vi "Master Setup Prompt.vi"(7 "Master Setup File (in)":path) -> (2 "Current File Paths":path[](array[path]), 3 "Master Setup File (out)":path)   [LabVIEW 2017]
panel:
  in  "Auto Correct":bool
  in  "Continue":bool
  in  "Clear Files":bool
  in  "Clear":bool[](array[boolean])
  out "Setup Description":string[](array[string])
  in  "Browse":bool[](array[boolean])
  in  "Select Directory":bool
  in  "Cancel":bool
  in  "OK":bool
  out "Status":u16[](array[ring])
  out "Old File Paths":path[](array[path])
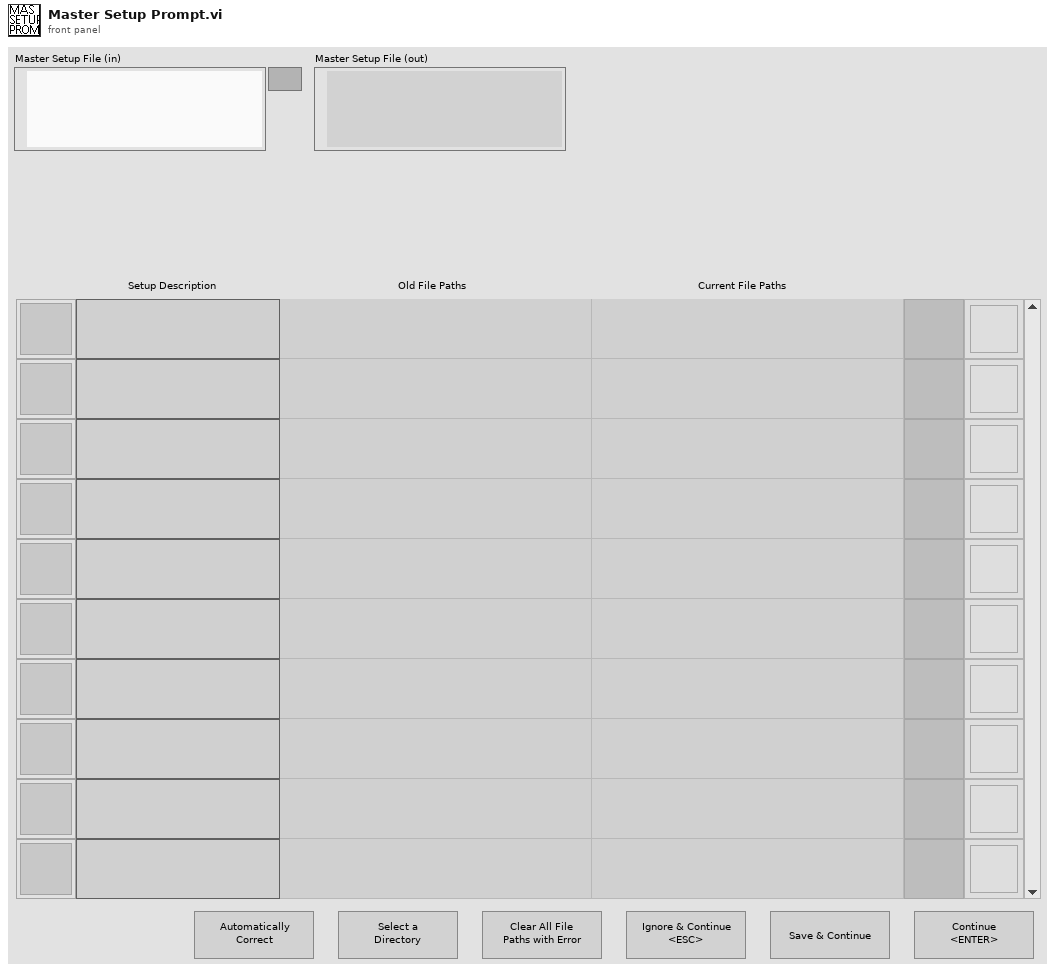
[diagram p1: front panel]
types:
  T1 = enum16{"Initialize", "Load Master Setup", "Check if Files Exist", "Idle", "Automatically Correct", "Browse for Directory", "Clear Files with Error", "Browse for File", "Clear Selected File", "Save Changes"}
  T2 = enum16{"open", "replace", "create", "open or create", "replace or create", "replace or create with confirmation"}
  T3 = enum16{"Initialize", "Load Master Setup", "Check if Files Exist", "Idle", "Automatically Correct", "Browse for Directory", "Clear Files with Error", "Browse for File", "Clear Selected File", "Save Changes"}[]
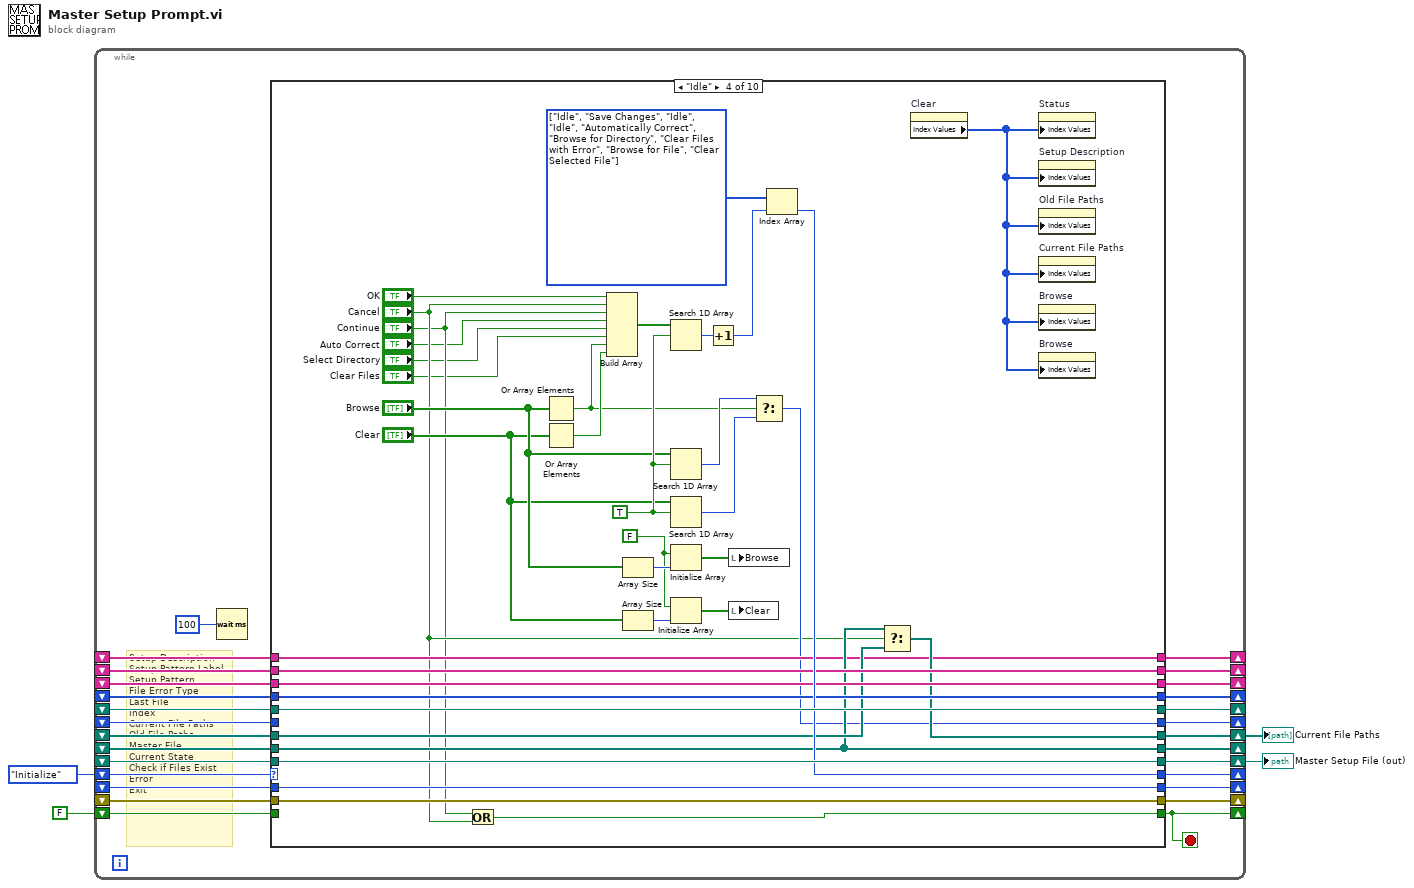
[diagram p0: block diagram]
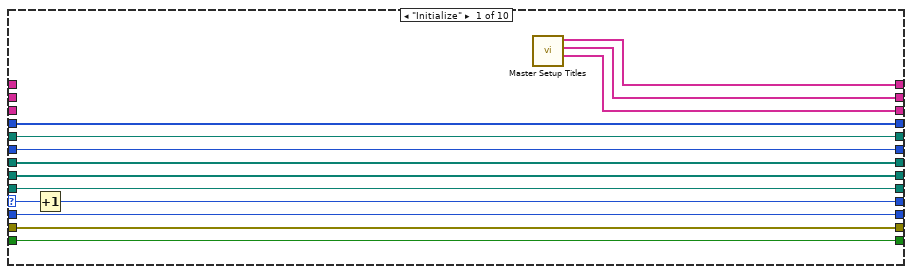
[diagram p2: hidden frame]
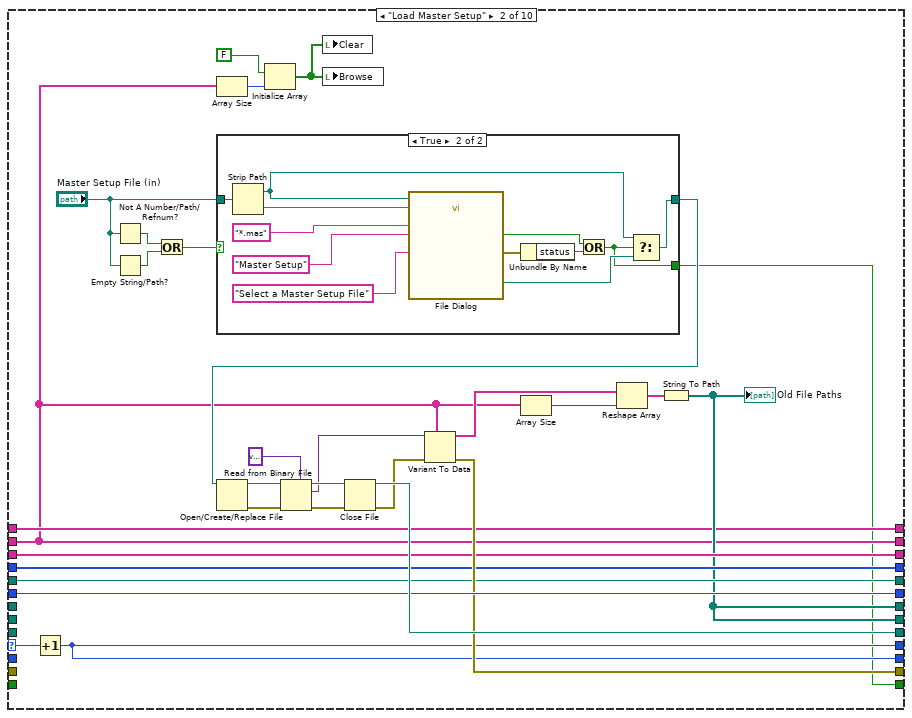
[diagram p3: hidden frame]
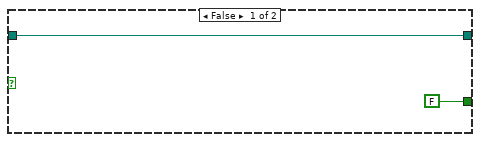
[diagram p4: hidden frame]
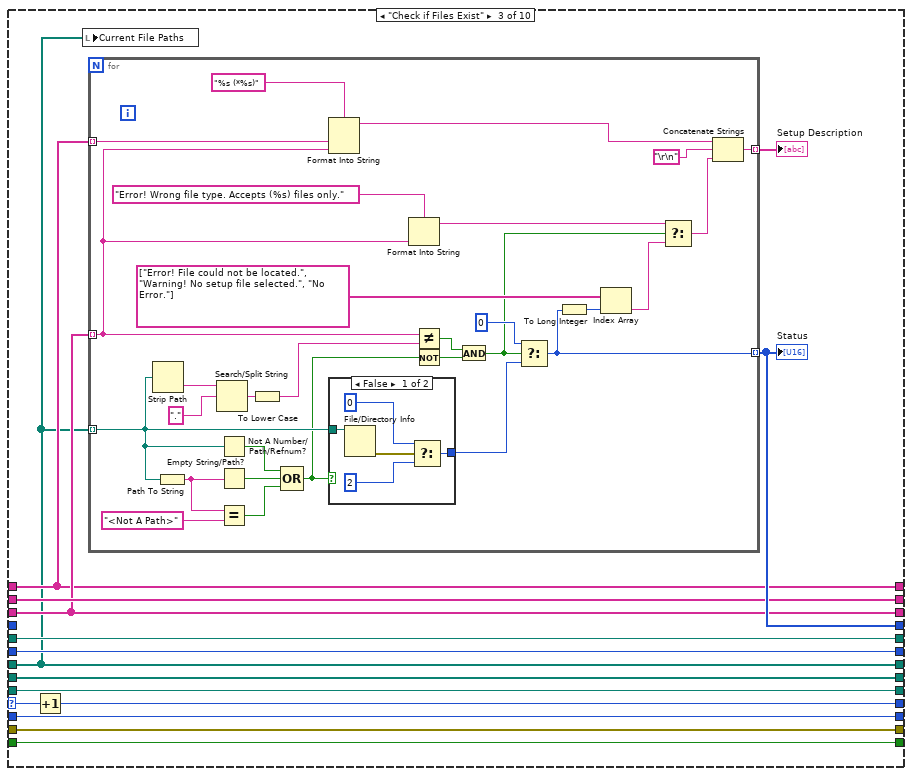
[diagram p5: hidden frame]
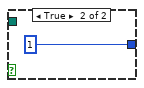
[diagram p6: hidden frame]
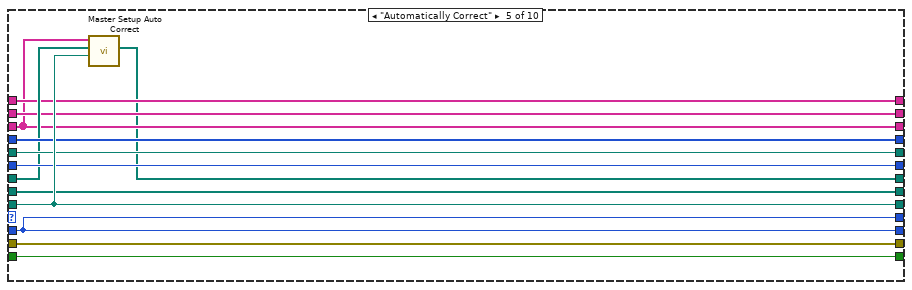
[diagram p7: hidden frame]
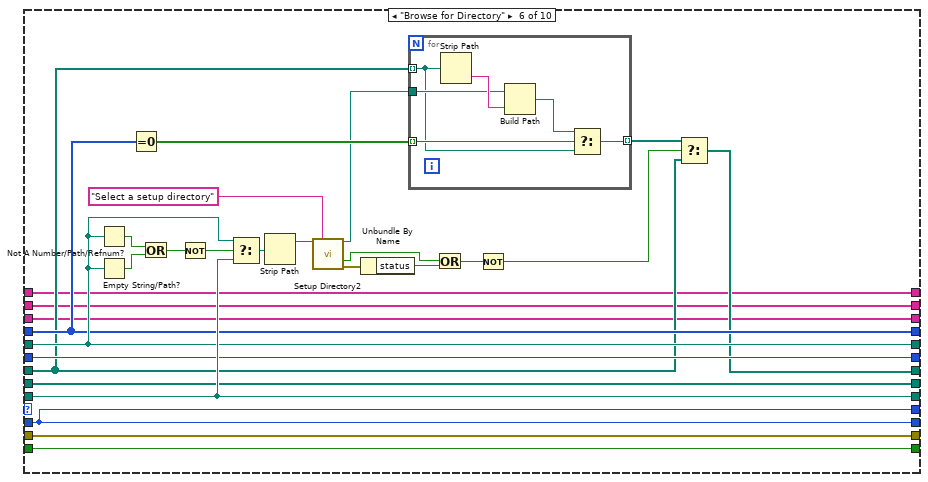
[diagram p8: hidden frame]
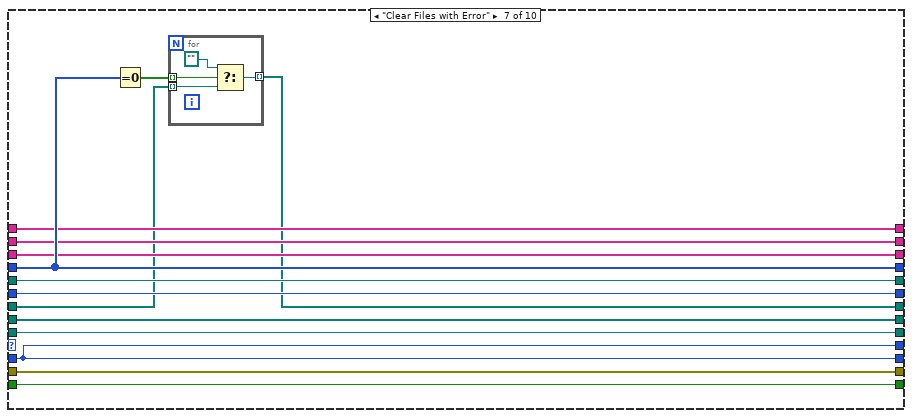
[diagram p9: hidden frame]
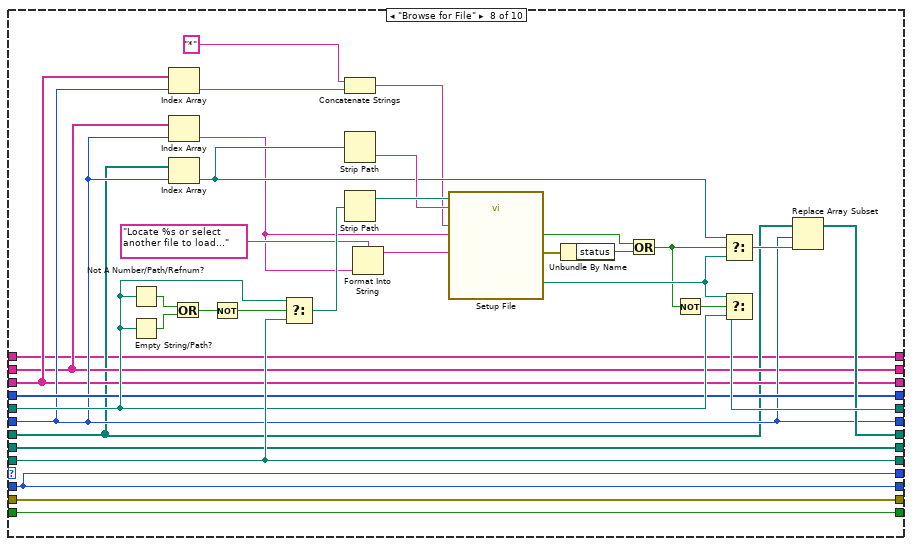
[diagram p10: hidden frame]
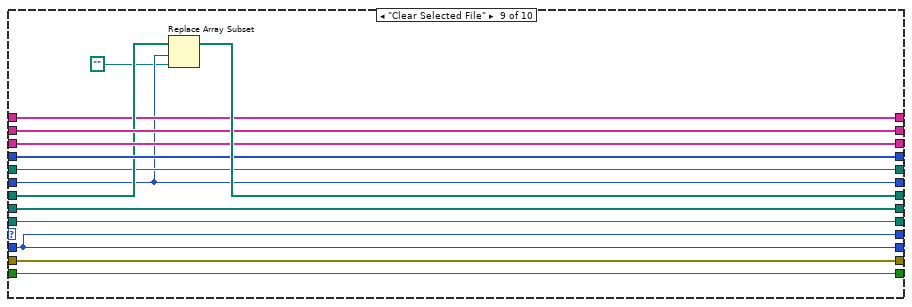
[diagram p11: hidden frame]
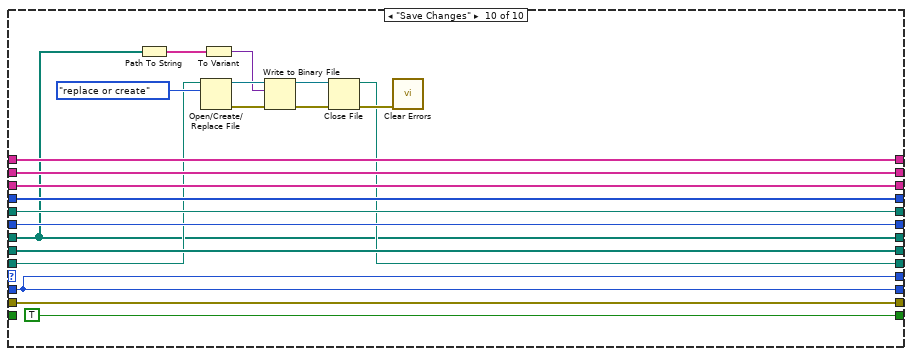
[diagram p12: hidden frame]
diagram:
  n1 = while {
    shift-right: [w21] -> _
    shift-left: FALSE -> [w25]
    shift-right: [w30] -> w3
    shift-left: _ -> [w31]
    shift-right: [w28] -> _
    shift-left: _ -> [w29]
    shift-right: [w26] -> w2
    shift-left: _ -> [w27]
    shift-right: [w18] -> _
    shift-left: T1."Initialize" -> [w24]
    shift-right: [w22] -> _
    shift-left: _ -> [w23]
    shift-right: [w19] -> _
    shift-left: _ -> [w20]
    shift-right: [w16] -> _
    shift-left: _ -> [w17]
    shift-right: [w13] -> _
    shift-left: _ -> [w14]
    shift-right: [w9] -> _
    shift-left: _ -> [w12]
    shift-right: [w10] -> _
    shift-left: _ -> [w11]
    shift-right: [w7] -> _
    shift-left: _ -> [w8]
    shift-right: [w5] -> _
    shift-left: _ -> [w6]
    stop <- w21 stop-if-true
    # "Setup Description\nSetup Pattern Label\nSetup Pattern\nFile Error Type\nLast File\nIndex\nCurrent File Paths\nOld File Paths\nMaster File\nCurrent State\nCheck if Files Exist\nError\nExit"
    n2 = Wait (ms)(milliseconds to wait=u32 100) -> ()  [unwired: 1 out]
    n3 = case shown="\"Idle\"" w24 {
      selector: w24 -> [w42 w64 w101 _ _ _ _ _ _ _]
      tunnel: w25 -> [w45 _ w100 _ w187 w206 w235 w257 w288 _]
      tunnel: w31 -> [w41 _ w103 w175 w188 w208 w236 w266 w289 w294]
      tunnel: [w45 w47 w100 w145 w187 w206 w235 w257 w288 TRUE] -> w21
      tunnel: [w41 w71 w103 w175 w188 w208 w236 w266 w289 w293] -> w30
      tunnel: w29 -> [w44 _ w104 w176 w189 w217 w237 w276 w290 w311]
      tunnel: [w44 w66 w104 w176 w189 w217 w237 w276 w290 w311] -> w28
      tunnel: w27 -> [w40 _ w90 w163 w182 w195 w225 w246 w282 w292]
      tunnel: [w40 w58 w90 w161 w177 w194 w224 w254 w286 w292] -> w26
      tunnel: w23 -> [w39 w67 w99 _ w185 w204 w233 w251 w278 w310]
      tunnel: [w36 w63 w98 w169 w186 w205 w234 w256 w287 w309] -> w18
      tunnel: [w39 w67 w99 w156 w185 w204 w233 w251 w278 w310] -> w22
      tunnel: w20 -> [w38 w65 w102 w174 w184 w202 w232 w262 w279 w308]
      tunnel: [w38 w65 w102 w174 w184 w202 w232 w255 w279 w308] -> w19
      tunnel: w17 -> [w43 _ w97 w168 w186 w205 w234 w256 w287 w309]
      tunnel: [w43 w63 w97 w168 w186 w205 w234 w256 w287 w309] -> w16
      tunnel: w14 -> [w37 w60 _ w166 w183 w201 w231 w252 w285 w306]
      tunnel: [w37 w60 w96 w166 w183 w201 w231 w252 w285 w306] -> w13
      tunnel: w12 -> [_ w59 w93 w165 w178 w192 w228 w248 w284 w305]
      tunnel: w11 -> [_ w49 w95 w164 w181 w193 w229 w247 w283 w304]
      tunnel: [w33 w49 w95 w164 w181 w193 w229 w247 w283 w304] -> w10
      tunnel: [w32 w59 w93 w165 w178 w192 w228 w248 w284 w305] -> w9
      tunnel: w8 -> [w35 _ w94 w162 w180 w191 w227 w245 w281 w303]
      tunnel: [w35 w58 w94 w162 w180 w191 w227 w245 w281 w303] -> w7
      tunnel: w6 -> [_ w52 w92 w160 w179 w190 w226 w244 w280 w302]
      tunnel: [w34 w52 w92 w160 w179 w190 w226 w244 w280 w302] -> w5
      frame "Initialize" {
        n4 = Increment(x=w42) -> (x+1=w36:T1)
        n5 = call "Master Setup Titles.vi"() -> ("Setup Patterns"=w32:string[], "Setup Description"=w33:string[], "Setup Description w/Numbers"=w34:string[])  [unwired: 6 in, 3 out]
      }
      frame "Load Master Setup" {
        n6 = Increment(x=w64) -> (x+1=w63:T1)
        n7 = Not A Number/Path/Refnum?(number/path/refnum="Master Setup File (in)") -> (NaN/Path/Refnum?=w57:bool)
        n8 = Empty String/Path?(string/path="Master Setup File (in)") -> (empty?=w56:bool)
        n9 = Or(x=w57, y=w56) -> (x .or. y?=w55:bool)
        n10 = Array Size(array=w49) -> (size(s)=w62:i32)
        n11 = case shown="True" w55 {
          tunnel: "Master Setup File (in)" -> [w77 w89]
          tunnel: [w77 w80] -> w53
          tunnel: [FALSE w79] -> w47
          frame False {
          }
          frame True {
            n12 = Strip Path(path=w89) -> (stripped path=w78:path, name=w88:string)
            n13 = call "File Dialog"("start path"=w78, "prompt"="Select a Master Setup File", "default name"=w88, "pattern (all files)"="*.mas", "pattern label"="Master Setup") -> ("selected path"=w81:path, "cancelled"=w82:bool, "error out"=w84:errorcluster)  [unwired: 7 in, 1 out]
            n14 = Unbundle By Name(w84) -> ("status"=w83:bool)
            n15 = Or(x=w82, y=w83) -> (x .or. y?=w79:bool)
            n16 = Select(t=w78, s=w79, f=w81) -> (s? t:f=w80:path)
          }
        }
        n17 = Open/Create/Replace File(file path (use dialog)=w53) -> (refnum out=w73:refnum<file>, error out=w75:errorcluster)  [unwired: 5 in, 1 out]
        n18 = Initialize Array(FALSE, w62) -> (w46:bool[])
        n19 = Read from Binary File(5:variant ("Data (in)"), 8:w75, 11:w73) -> (0:w74:errorcluster, 2:w69:variant, 3:w72:refnum<file>)  [unwired: 3 in, 1 out]
        n20 = local write "Clear"(w46) -> ()
        n21 = local write "Browse"(w46) -> ()
        n22 = Close File(refnum=w72, error in=w74) -> (path=w71:path, error out=w68:errorcluster)
        n23 = Variant To Data(error in=w68, type=w49, Variant=w69) -> (data=w51:string[], error out=w66:errorcluster)
        n24 = Array Size(array=w49) -> (size(s)=w50:i32)
        n25 = Reshape Array(w51, w50) -> (w48:string[])
        n26 = String To Path(string=w48) -> (path=w58:path[])
        "Old File Paths" <- w58
      }
      frame "Check if Files Exist" {
        n27 = Increment(x=w101) -> (x+1=w98:T1)
        n28 = local write "Current File Paths"(w90) -> ()
        n29 = for {
          tunnel: w90 -> [w128] mode=indexing
          tunnel: [w122] -> w96 mode=indexing
          tunnel: w93 -> [w106] mode=indexing
          tunnel: w92 -> [w108] mode=indexing
          tunnel: [w116] -> w91 mode=indexing
          n30 = Strip Path(path=w128) -> (name=w127:string)  [unwired: 1 out]
          n31 = Path To String(path=w128) -> (string=w131:string)
          n32 = Search/Split String(string=w127, search string/char (-)=".") -> (match + rest of string=w117:string)  [unwired: 1 in, 2 out]
          n33 = Not A Number/Path/Refnum?(number/path/refnum=w128) -> (NaN/Path/Refnum?=w132:bool)
          n34 = Empty String/Path?(string/path=w131) -> (empty?=w133:bool)
          n35 = Equal?(x=w131, y="<Not A Path>") -> (x = y?=w129:bool)
          n36 = To Lower Case(string=w117) -> (all lower case string=w109:string)
          n37 = Compound Arithmetic op=OR(w132, w133, w129) -> (w111:bool)
          n38 = Format Into String(format string="%s (*%s)" ("search string/char (-)"), w108, w106) -> (resulting string=w107:string)  [unwired: 2 in, 1 out]
          n39 = case shown="False" w111 {
            tunnel: w128 -> [w138 _]
            tunnel: [w134 u16 1] -> w125
            frame False {
              n40 = File/Directory Info(path=w138) -> (error out=w137:errorcluster)  [unwired: 1 in, 6 out]
              n41 = Select(t=u16 0, s=w137, f=u16 2) -> (s? t:f=w134:u16)
            }
            frame True {
            }
          }
          n42 = Format Into String(format string="Error! Wrong file type. Accepts (%s) files only.", w106) -> (resulting string=w119:string)  [unwired: 2 in, 1 out]
          n43 = Not Equal?(x=w106, y=w109) -> (x != y?=w112:bool)
          n44 = Not(x=w111) -> (.not. x?=w110:bool)
          n45 = And(x=w112, y=w110) -> (x .and. y?=w113:bool)
          n46 = Select(t=u16 0, s=w113, f=w125) -> (s? t:f=w122:u16)
          n47 = To Long Integer(number=w122) -> (32bit integer=w121:i32)
          n48 = Index Array(array=string[] ["Error! File could not be located.", "Warning! No setup file selected.", "No Error."], index=w121) -> (element=w120:string)
          n49 = Select(t=w119, s=w113, f=w120) -> (s? t:f=w115:string)
          n50 = Concatenate Strings(w107, "\r\n", w115) -> (w116:string)
        }
        "Status" <- w96
        "Setup Description" <- w91
      }
      frame "Idle" {
        w147 = T3 [enum."Idle", enum."Save Changes", enum."Idle", enum."Idle", enum."Automatically Correct", enum."Browse for Directory", enum."Clear Files with Error", enum."Browse for File", enum."Clear Selected File"] items=["Initialize", "Load Master Setup", "Check if Files Exist", "Idle", "Automatically Correct", "Browse for Directory", "Clear Files with Error", "Browse for File", "Clear Selected File", "Save Changes"]
        w152 = FALSE
        w159 = TRUE ("element")
        n51 = Or(x="Continue", y="Cancel") -> (x .or. y?=w145:bool)
        n52 = Or Array Elements(Boolean array="Browse") -> (logical OR=w148:bool)
        n53 = Or Array Elements(Boolean array="Clear") -> (logical OR=w149:bool)
        n54 = Build Array("OK", "Cancel", "Continue", "Auto Correct", "Select Directory", "Clear Files", w148, w149) -> (w172:bool[])
        n55 = Array Size(array="Browse") -> (size(s)=w154:i32)
        n56 = Array Size(array="Clear") -> (size(s)=w153:i32)
        n57 = Search 1D Array(1D array=w172, element=w159) -> (index of element=w171:i32)  [unwired: 1 in]
        n58 = Search 1D Array(1D array="Browse", element=w159) -> (index of element=w158:i32)  [unwired: 1 in]
        n59 = Search 1D Array(1D array="Clear", element=w159) -> (index of element=w157:i32)  [unwired: 1 in]
        n60 = Initialize Array(w152, w154) -> (w167:bool[])
        n61 = Initialize Array(w152, w153) -> (w150:bool[])
        n62 = Increment(x=w171) -> (x+1=w170:i32)
        n63 = local write "Browse"(w167) -> ()
        n64 = local write "Clear"(w150) -> ()
        n65 = Select(t=w158, s=w148, f=w157) -> (s? t:f=w156:i32)
        n66 = Index Array(array=w147, index=w170) -> (element=w169:T1)
        n67 = Select(t=w162, s="Cancel", f=w163) -> (s? t:f=w161:path[])
        n68 = property on="Clear" class="Arr"() -> ("Index Values"=w146:u32[])  [unwired: 2 in, 2 out]
        n69 = property on="Status" class="Arr (strict)"("Index Values"=w146) -> ()  [unwired: 2 in, 2 out]
        n70 = property on="Setup Description" class="Arr (strict)"("Index Values"=w146) -> ()  [unwired: 2 in, 2 out]
        n71 = property on="Old File Paths" class="Arr (strict)"("Index Values"=w146) -> ()  [unwired: 2 in, 2 out]
        n72 = property on="Current File Paths" class="Arr (strict)"("Index Values"=w146) -> ()  [unwired: 2 in, 2 out]
        n73 = property on="Browse" class="Arr"("Index Values"=w146) -> ()  [unwired: 2 in, 2 out]
        n74 = property on="Browse" class="Arr"("Index Values"=w146) -> ()  [unwired: 2 in, 2 out]
      }
      frame "Automatically Correct" {
        n75 = call "Master Setup Auto Correct.vi"("Master File Path"=w188, "Current File Paths (in)"=w182, "Setup Patterns"=w178) -> ("Current File Paths (out)"=w177:path[])  [unwired: 8 in]
      }
      frame "Browse for Directory" {
        n76 = Not A Number/Path/Refnum?(number/path/refnum=w202) -> (NaN/Path/Refnum?=w212:bool)
        n77 = Empty String/Path?(string/path=w202) -> (empty?=w211:bool)
        n78 = Equal To 0?(x=w201) -> (x = 0?=w200:bool[])
        n79 = Or(x=w212, y=w211) -> (x .or. y?=w210:bool)
        n80 = Not(x=w210) -> (.not. x?=w209:bool)
        n81 = Select(t=w202, s=w209, f=w208) -> (s? t:f=w207:path)
        n82 = Strip Path(path=w207) -> (stripped path=w216:path)  [unwired: 1 out]
        n83 = call "Setup Directory2"("start path"=w216, "prompt"="Select a setup directory") -> ("selected path"=w199:path, "cancelled"=w213:bool, "error out"=w215:errorcluster)  [unwired: 10 in, 1 out]
        n84 = Unbundle By Name(w215) -> ("status"=w214:bool)
        n85 = for {
          tunnel: w200 -> [w223] mode=indexing
          tunnel: w195 -> [w219] mode=indexing
          tunnel: w199 -> [w221]
          tunnel: [w218] -> w196 mode=indexing
          n86 = Strip Path(path=w219) -> (name=w222:string)  [unwired: 1 out]
          n87 = Build Path(base path=w221, name or relative path=w222) -> (appended path=w220:path)
          n88 = Select(t=w220, s=w223, f=w219) -> (s? t:f=w218:path)
        }
        n89 = Or(x=w213, y=w214) -> (x .or. y?=w198:bool)
        n90 = Not(x=w198) -> (.not. x?=w197:bool)
        n91 = Select(t=w196, s=w197, f=w195) -> (s? t:f=w194:path[])
      }
      frame "Clear Files with Error" {
        n92 = Equal To 0?(x=w231) -> (x = 0?=w230:bool[])
        n93 = for {
          tunnel: w230 -> [w241] mode=indexing
          tunnel: w225 -> [w240] mode=indexing
          tunnel: [w239] -> w224 mode=indexing
          n94 = Select(t=path "", s=w241, f=w240) -> (s? t:f=w239:path)
        }
      }
      frame "Browse for File" {
        n95 = Not A Number/Path/Refnum?(number/path/refnum=w262) -> (NaN/Path/Refnum?=w271:bool)
        n96 = Empty String/Path?(string/path=w262) -> (empty?=w270:bool)
        n97 = Index Array(array=w248, index=w251) -> (element=w250:string)
        n98 = Index Array(array=w247, index=w251) -> (element=w249:string)
        n99 = Index Array(array=w246, index=w251) -> (element=w253:path)
        n100 = Or(x=w271, y=w270) -> (x .or. y?=w269:bool)
        n101 = Not(x=w269) -> (.not. x?=w268:bool)
        n102 = Select(t=w262, s=w268, f=w266) -> (s? t:f=w265:path)
        n103 = Concatenate Strings("*" ("string"), w250) -> (w243:string)
        n104 = Strip Path(path=w253) -> (name=w258:string)  [unwired: 1 out]
        n105 = Strip Path(path=w265) -> (stripped path=w275:path)  [unwired: 1 out]
        n106 = Format Into String(format string="Locate %s or select another file to load..." ("prompt"), w249) -> (resulting string=w260:string)  [unwired: 2 in, 1 out]
        n107 = call "Setup File"("start path"=w275, "prompt"=w260, "default name"=w258, "pattern (all files)"=w243, "pattern label"=w249) -> ("selected path"=w264:path, "cancelled"=w272:bool, "error out"=w274:errorcluster)  [unwired: 7 in, 1 out]
        n108 = Unbundle By Name(w274) -> ("status"=w273:bool)
        n109 = Or(x=w272, y=w273) -> (x .or. y?=w263:bool)
        n110 = Not(x=w263) -> (.not. x?=w261:bool)
        n111 = Select(t=w253, s=w263, f=w264) -> (s? t:f=w267:path)
        n112 = Select(t=w264, s=w261, f=w262) -> (s? t:f=w255:path)
        n113 = Replace Array Subset(array=w246, new element=w267, index=w251) -> (w254:path[])
      }
      frame "Clear Selected File" {
        n114 = Replace Array Subset(array=w282, new element=path "", index=w278) -> (w286:path[])
      }
      frame "Save Changes" {
        n115 = Path To String(path=w292) -> (string=w291:string[])
        n116 = Open/Create/Replace File(file path (use dialog)=w294, operation (0:open)=T2."replace or create") -> (refnum out=w301:refnum<file>, error out=w299:errorcluster)  [unwired: 4 in, 1 out]
        n117 = To Variant(anything=w291) -> (Variant=w296:variant)
        n118 = Write to Binary File(file (use dialog)=w301, data=w296, error in=w299) -> (refnum out=w300:refnum<file>, error out=w298:errorcluster)  [unwired: 3 in, 1 out]
        n119 = Close File(refnum=w300, error in=w298) -> (path=w293:path, error out=w295:errorcluster)
        n120 = call <vilib>:"Clear Errors.vi"("error in (no error)"=w295) -> ()  [unwired: 5 in, 2 out]
      }
    }
  }
  "Master Setup File (out)" <- w3
  "Current File Paths" <- w2
